vi "_Main.vi"   [LabVIEW 2016, in "WC_Drive.lvlib"]
uses:
  WC_Drive.lvlib
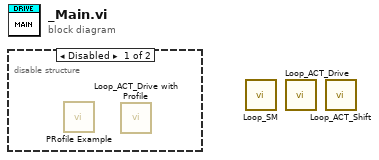
[diagram p0: block diagram]
diagram:
  n1 = disable-structure shown="Disabled" {
    frame Disabled {
      n2 = call "PRofile Example.vi"() -> ()  [unwired: 12 in]
      n3 = call "Loop_ACT_Drive with Profile.vi"() -> ()  [unwired: 12 in]
    }
    frame Enabled {
    }
  }
  n4 = call "Loop_SM.vi"() -> ()  [unwired: 12 in]
  n5 = call "Loop_ACT_Drive.vi"() -> ()  [unwired: 12 in]
  n6 = call "Loop_ACT_Shift.vi"() -> ()  [unwired: 12 in]
